vi "RichToFlatgrpc_reflection_v1alpha_ExtensionRequest.vi"(5 "OutputClusterType":T1, 11 "InputCluster":T2) -> (3 "OutputCluster":T1)   [LabVIEW 2025, in "reflection_client.lvlib"]
uses:
  reflection_client.lvlib
  grpc_reflection_v1alpha_ExtensionRequest.ctl
  grpc_reflection_v1alpha_ExtensionRequest_Flat.ctl
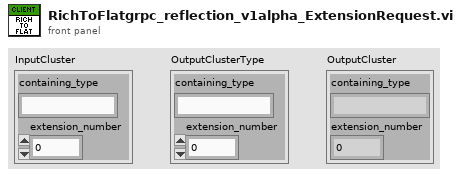
[diagram p1: front panel]
types:
  T1 = typedef "reflection_client.lvlib/grpc_reflection_v1alpha_ExtensionRequest_Flat.ctl" = cluster{"containing_type":string, "extension_number":i32}
  T2 = typedef "reflection_client.lvlib/grpc_reflection_v1alpha_ExtensionRequest.ctl" = cluster{"containing_type":string, "extension_number":i32}
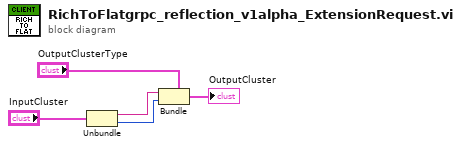
[diagram p0: block diagram]
diagram:
  n1 = Unbundle "Unbundle"("InputCluster") -> ("containing_type"=w2:string, "extension_number"=w1:i32)
  n2 = Bundle "Bundle"(cluster="OutputClusterType", "containing_type"=w2, "extension_number"=w1) -> (→"OutputCluster":T1)
